vi "PCO_SetSensorFormat.vi"(8 "error in (no error)":errorcluster {"code" format="%x"}, 10 "wSensor":u16(ring) items=["standard", "extended"], 11 "ph":u64) -> (0 "error out":errorcluster {"code" format="%x"}, 2 "ErrorMessage":i32 format="%x", 3 "ph out":u64)   [LabVIEW 2020, in "SDK.lvlib" / "ImageSensor.lvlib"]
doc: "<b>Description:</b>\nThis function does set the sensor format. In the format [standard] only effective pixels are readout from the sensor. The readout in the format [extended] is camera dependent. Either a distinct region of the sensor is selected or the full sensor including effective, dark, reference and dummy pixels. Invalid values result in a failure response message.\nThe command will be rejected, if Recording State is [run], see PCO_GetRecordingState.\n\n<b>Supported camera type:</b>\nAll cameras\n\n<b>Descriptor dependency:</b>\nNone"
uses:
  ImageSensor.lvlib
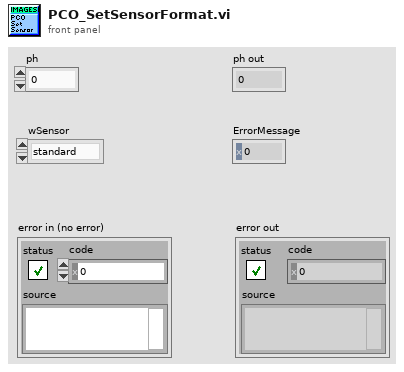
[diagram p1: front panel]
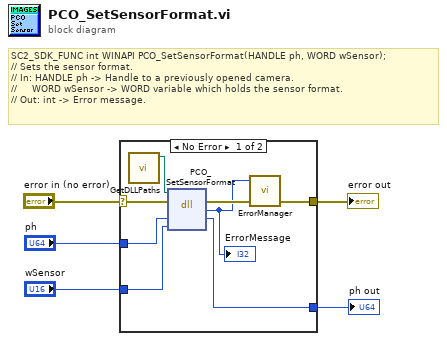
[diagram p0: block diagram]
diagram:
  # "SC2_SDK_FUNC int WINAPI PCO_SetSensorFormat(HANDLE ph, WORD wSensor);\n// Sets the sensor format.\n// In: HANDLE ph -> Handle to a previously opened camera.\n//     WORD wSensor -> WORD variable which holds the sensor format.\n// Out: int -> Error message."
  n1 = case shown="No Error" "error in (no error)" {
    selector: "error in (no error)" -> [w10 w15]
    tunnel: "ph" -> [w13 w14]
    tunnel: [w12 w14] -> w4
    tunnel: "wSensor" -> [w11 _]
    tunnel: [w8 w15] -> w2
    frame No Error {
      n2 = call "GetDLLPaths.vi"() -> ("SC2_Cam_Path"=w6:path)  [unwired: 9 in, 2 out]
      n3 = dll-call lib="F:/DKI/LabView/LabView/LabView_SDK/SC2_Cam.*" fn="PCO_SetSensorFormat"(path in=w6, error in=w10, "ph"=w13, "wSensor"=w11) -> (error out=w9:errorcluster, "return type"=w7:i32, "ph"=w12:u64)  [unwired: 2 in, 1 out]
      "ErrorMessage" <- w7
      n4 = call "ErrorManager.vi"("error in (no error)"=w9, "error code"=w7) -> ("error out"=w8:errorcluster)  [unwired: 3 in]
    }
    frame Error {
    }
  }
  "ph out" <- w4
  "error out" <- w2
